vi "GoAndTakePic.vi"() -> ()   [LabVIEW 2021]
uses:
  <vilib>/userDefined/High Color/IMAQdx.ctl
  <vilib>/Utility/file.llb/Read Delimited Spreadsheet (DBL).vi
  <vilib>/vision/driver/NI_Vision_Acquisition_Software.lvlib
panel:
  in  "Camera":T1="cam1"
  out "BestZvalue":dbl
  in  "AbortAutoFocus":bool
  out "N_iterations":dbl[](array[numeric])
  out "UsedCoordinates":string
  in  "ImageName":string="Image"
  out "error out":errorcluster
  in  "OutImagePath":string="C:\\Users\\TTUHEP\\Pictures\\GantryCamGoTakePic\\"
  in  "AutoFocus":bool
  in  "SafeMaxZ":dbl=75.0 format="%#_13g"
  out "Image":T2(plugin-control)
  in  "Zoffset_textFile":dbl
  in  "Positions":path=path "C:/Users/TTUHEP/Documents/LabVIEW/GantryPrograms/Configs/A1_BP_HeightMeasure.txt"
  in  "error in (no error)":errorcluster
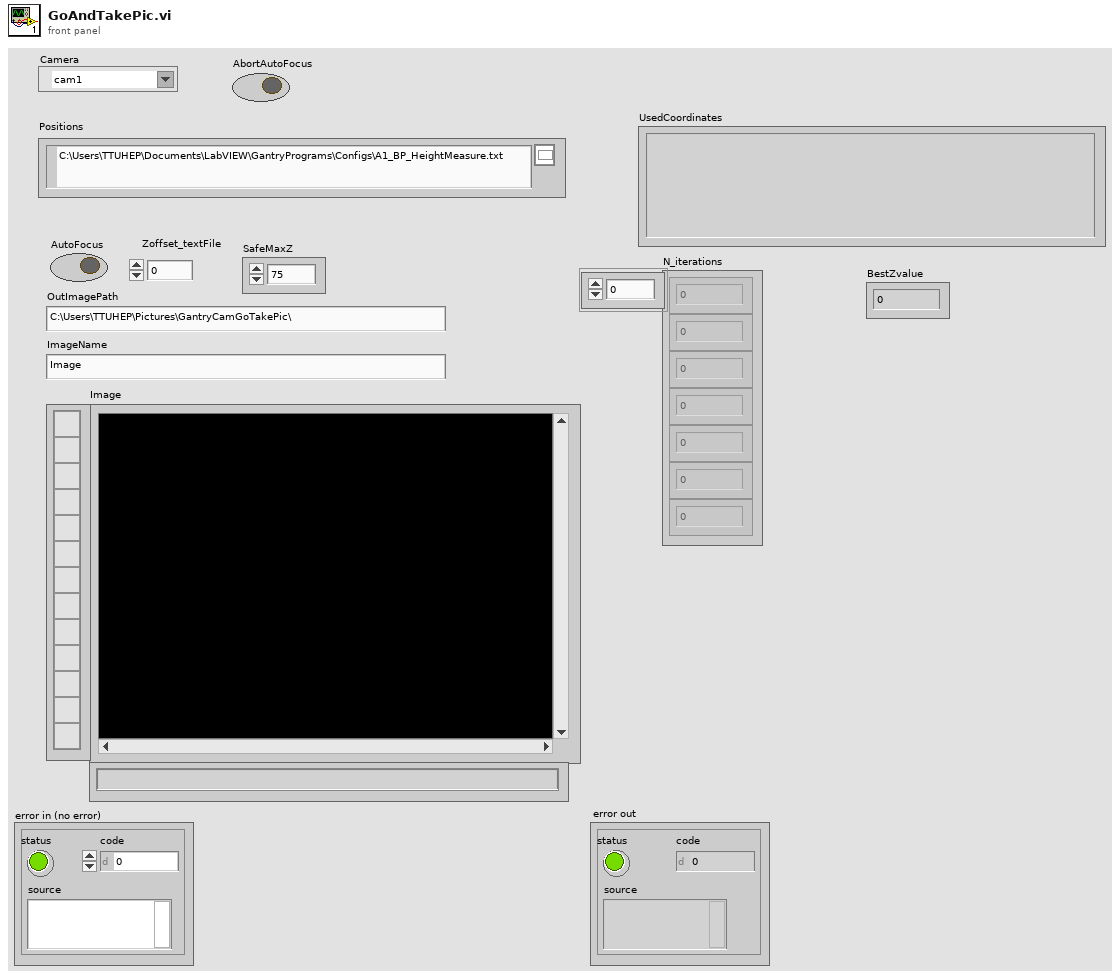
[diagram p1: front panel]
types:
  T1 = typedef "IMAQdx.ctl" = refnum<k21>
  T2 = typedef "IMAQ Image.ctl" = refnum<image>
  T3 = typedef "Image Type" = u32
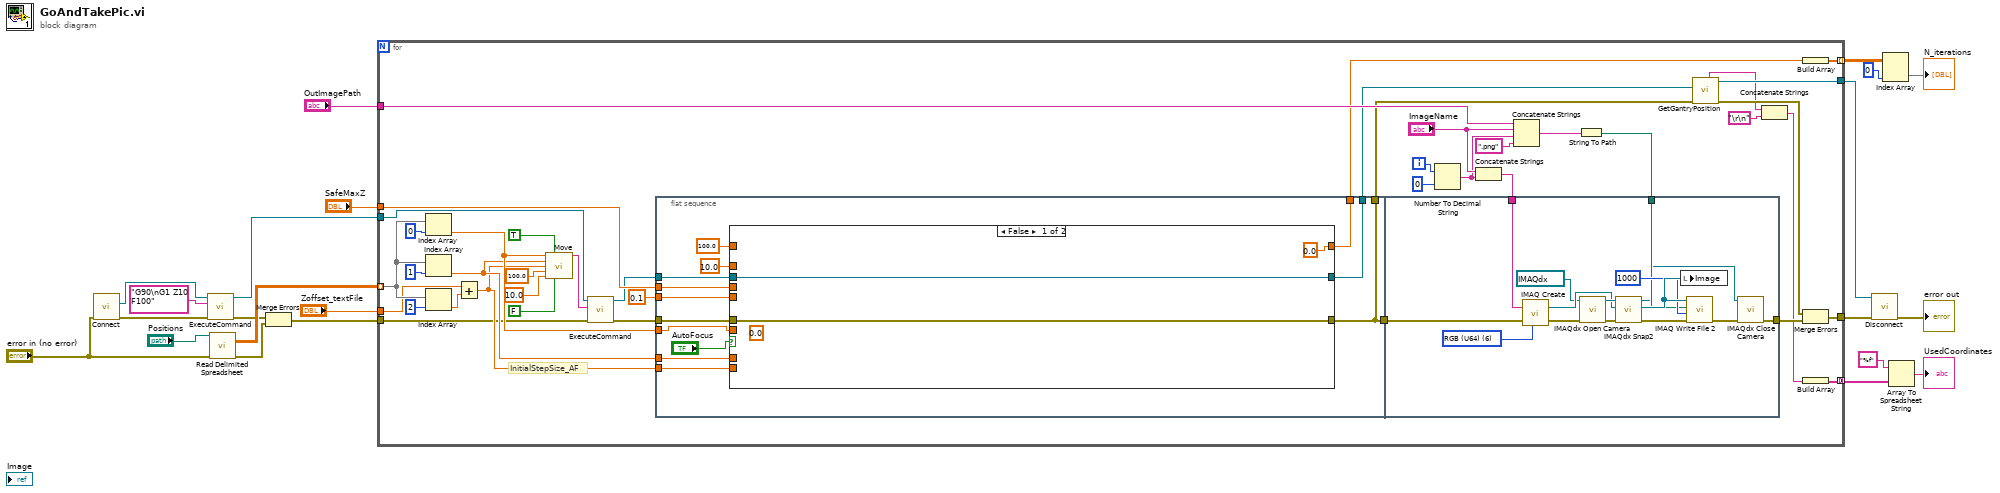
[diagram p0: block diagram]
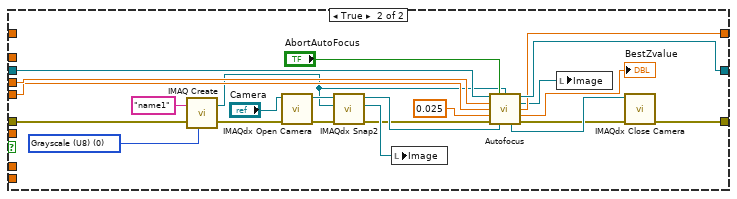
[diagram p2: hidden frame]
diagram:
  n1 = call "Connect.vi"("error in (no error)"="error in (no error)") -> ("error out"=w16:errorcluster, "controller"=w18:refnum<k24>)  [unwired: 9 in]
  n2 = call "ExecuteCommand.vi"("error in (no error)"=w16, "Command Code"="G90\nG1 Z10 F100", "controller in"=w18) -> ("error out"=w12:errorcluster, "controller out"=w15:refnum<k24>)  [unwired: 6 in, 1 out]
  n3 = call-poly <vilib>:"Read Delimited Spreadsheet.vi"("file path (dialog if empty)"="Positions", "error in (no error)"="error in (no error)") -> ("all rows"=w22:dbl[][], "error out"=w11:errorcluster)  [unwired: 8 in, 4 out]
  n4 = Merge Errors(w12, w11) -> (w2:errorcluster)
  n5 = for {
    tunnel: w22 -> [w61] mode=indexing
    tunnel: w2 -> [w46]
    tunnel: [w28] -> w6 mode=indexing
    tunnel: w15 -> [w49]
    tunnel: "SafeMaxZ" -> [w59]
    tunnel: "Zoffset_textFile" -> [w58]
    tunnel: [w31] -> w3
    tunnel: [w29] -> w9 mode=concatenating
    tunnel: [w35] -> w13
    tunnel: "OutImagePath" -> [w44]
    i -> [w43]
    # "InitialStepSize_AF"
    n6 = Index Array(array=w61, index=0) -> (element=w56:dbl)
    n7 = Index Array(array=w61, index=1) -> (element=w55:dbl)
    n8 = Index Array(array=w61, index=2) -> (element=w57:dbl)
    n9 = Add(x=w58, y=w57) -> (x+y=w54:dbl)
    n10 = call "Move.vi"("X"=w56, "Absolute"=TRUE, "Y"=w55, "Z"=w54, "SpeedXY (mm/s)"=100.0, "SpeedZ (mm/s)"=10.0, "Move Z first"=FALSE) -> ("Position Gcode"=w47:string)  [unwired: 8 in]
    n11 = call "ExecuteCommand.vi"("error in (no error)"=w46, "Command Code"=w47, "controller in"=w49) -> ("error out"=w45:errorcluster, "controller out"=w48:refnum<k24>)  [unwired: 6 in, 1 out]
    n12 = flat-sequence {
      tunnel: 0.1 ("InitialStepSize") -> [w77]
      tunnel: w59 -> [w74]
      tunnel: w56 -> [w73]
      tunnel: w55 -> [w72]
      tunnel: w54 -> [w71]
      tunnel: w48 -> [w70]
      tunnel: w45 -> [w69]
      tunnel: [w66] -> w37
      tunnel: [w67] -> w34
      tunnel: [w66] -> w30
      tunnel: [w65] -> w27
      tunnel: w37 -> [w112]
      tunnel: w36 -> [w110]
      tunnel: [w105] -> w32
      tunnel: w26 -> [w108]
      frame #0 {
        n13 = case shown="False" "AutoFocus" {
          tunnel: [w78 w95] -> w66
          tunnel: [w79 w103] -> w67
          tunnel: w77 -> [_ w98]
          tunnel: [0.0 ("N_iterations") w102] -> w65
          tunnel: 100.0 ("SpeedXY (mm/s)") -> [_ _]
          tunnel: 10.0 ("SpeedZ (mm/s)") -> [_ _]
          tunnel: w74 -> [_ w99]
          tunnel: w73 -> [_ _]
          tunnel: w72 -> [_ _]
          tunnel: w71 -> [_ _]
          tunnel: w70 -> [w79 w101]
          tunnel: w69 -> [w78 w82]
          frame False {
            (unwired) 0.0 ("BestZvalue")
          }
          frame True {
            w89 = T3 0 items=["Grayscale (U8)", "Grayscale (I16)", "Grayscale (SGL)", "Complex (CSG)", "RGB (U32)", "HSL (U32)", "RGB (U64)", "Grayscale (U16)"] ("Image Type")
            n14 = call "IMAQ Create"("Image Name"="name1" ("ImageName"), "Image Type"=w89, "error in (no error)"=w82) -> ("New Image"=w85:T2, "error out"=w91:errorcluster)  [unwired: 2 in]
            n15 = call <vilib>:"IMAQdx Open Camera.vi"("error in"=w91, "Session In"="Camera") -> ("error out"=w86:errorcluster, "Session Out"=w87:T1)  [unwired: 8 in]
            n16 = call <vilib>:"IMAQdx Snap2.vi"("error in"=w86, "Image In"=w85, "Session In"=w87) -> ("error out"=w81:errorcluster, "Image Out"=w83:T2, "Session Out"=w84:T1)  [unwired: 6 in]
            n17 = local write "Image"(w83) -> ()
            n18 = call "Autofocus.vi"("controller in"=w101, "AbortAutoFocus"="AbortAutoFocus", "ImageIn"=w85, "SafeMaxZ"=w99, "InitialStepSize"=w98, "Tolerance"=0.025, "error in (no error)"=w81, "SessionIn"=w84) -> ("controller out"=w103:refnum<k24>, "Image"=w93:T2, "N_iterations"=w102:dbl, "BestZvalue"=→"BestZvalue":dbl, "Session Out"=w96:T1, "error out"=w94:errorcluster)  [unwired: 2 in]
            n19 = local write "Image"(w93) -> ()
            n20 = call <vilib>:"IMAQdx Close Camera.vi"("error in"=w94, "Session In"=w96) -> ("error out"=w95:errorcluster)  [unwired: 9 in]
          }
        }
      }
      frame #1 {
        w109 = T3 6 items=["Grayscale (U8)", "Grayscale (I16)", "Grayscale (SGL)", "Complex (CSG)", "RGB (U32)", "HSL (U32)", "RGB (U64)", "Grayscale (U16)"] ("Image Type")
        n21 = call "IMAQ Create"("Image Name"=w108, "Image Type"=w109, "error in (no error)"=w112) -> ("New Image"=w113:T2, "error out"=w117:errorcluster)  [unwired: 2 in]
        n22 = call <vilib>:"IMAQdx Open Camera.vi"("error in"=w117, "Session In"=T1 "cam1") -> ("error out"=w118:errorcluster, "Session Out"=w116:T1)  [unwired: 8 in]
        n23 = call <vilib>:"IMAQdx Snap2.vi"("error in"=w118, "Image In"=w113, "Session In"=w116) -> ("error out"=w115:errorcluster, "Image Out"=w114:T2, "Session Out"=w107:T1)  [unwired: 6 in]
        n24 = local write "Image"(w114) -> ()
        n25 = call-poly "IMAQ Write File 2"("error in (no error)"=w115, "Image Quality"=u32 1000, "File Path"=w110, "Image"=w114) -> ("error out"=w106:errorcluster)  [unwired: 6 in, 1 out]
        n26 = call <vilib>:"IMAQdx Close Camera.vi"("error in"=w106, "Session In"=w107) -> ("error out"=w105:errorcluster)  [unwired: 9 in]
      }
    }
    n27 = Number To Decimal String(number=w43, width (-)=i16 0) -> (decimal integer string=w38:string)
    n28 = Concatenate Strings("ImageName", w38) -> (w26:string)
    n29 = Concatenate Strings(w44, "ImageName", w38, ".png" ("string")) -> (w40:string)
    n30 = String To Path(string=w40) -> (path=w36:path)
    n31 = call "GetGantryPosition.vi"("error in (no error)"=w30, "Controller In"=w34) -> ("error out"=w33:errorcluster, "controller out"=w35:refnum<k24>, "Position_XYZ"=w25:string)  [unwired: 3 in, 4 out]
    n32 = Concatenate Strings(w25, "\r\n") -> (w23:string)
    n33 = Build Array(w27) -> (w28:dbl[])
    n34 = Merge Errors(w33, w32) -> (w31:errorcluster)
    n35 = Build Array(w23) -> (w29:string[])
  }
  n36 = call "Disconnect.vi"("error in (no error)"=w3, "controller"=w13) -> ("error out"=→"error out":errorcluster)  [unwired: 9 in]
  n37 = Index Array(array=w6, index (col)=0 ("disabled index (col)")) -> (element=→"N_iterations":dbl[])  [unwired: 1 in]
  n38 = Array To Spreadsheet String(array=w9, 3:"%f" ("format string")) -> (spreadsheet string=→"UsedCoordinates":string)  [unwired: 1 in]
